vi "VGD ECL AHMI PF SubVI04.vi"(0 "SUPERIOR":T1, 1 "error in":errorcluster) -> (2 "Redondez":dbl, 3 "Analisis superior":T1(plugin-control), 4 "error out":errorcluster)   [LabVIEW 2020]
uses:
  <vilib>/vision/Image Controls.llb/IMAQ Image.ctl
  <vilib>/vision/Measure.llb/Edge Options.ctl
  <vilib>/vision/Measure.llb/Edge Polarity.ctl
  <vilib>/vision/NI_Vision_Development_Module.lvlib
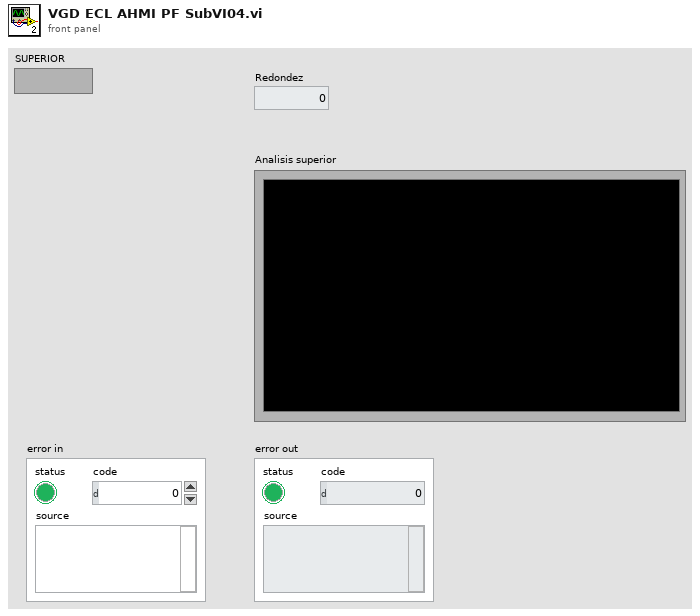
[diagram p1: front panel]
types:
  T1 = typedef "IMAQ Image.ctl" = refnum<image>
  T2 = typedef "Edge Options.ctl" = cluster{"Edge Polarity":T3, "Kernel Size":u32, "Width":u32, "Minimum Edge Strength":sgl, "Interpolation Type":enum32{"Zero Order", "Bilinear", "Quadratic", "Cubic", "Bilinear Fixed"}, "Data Processing Method":enum32{"Average", "Median"}}
  T3 = typedef "Edge Polarity.ctl" = u32
  T4 = cluster{"Search  Direction":u32, "Edge Options":T2, "Show Search Area":bool, "Show Search Lines":bool, "Show Edges Found":bool, "Show Result":bool, "Search Area Color":u32, "Search Lines Color":u32, "Edge Locations Color":u32, "Result Color":u32, "Overlay Group Name":string}
  T5 = cluster{"Process":enum16{"Get First Edge", "Get First + Last Edge", "Get All Edges", "Get Best Edge"}, "Step Size":dbl, "Max Pixel Radius":i32}
  T6 = typedef "IMAQ Circle" = cluster{"Center X":i32, "Center Y":i32, "Inner Radius":i32, "Outer Radius":i32, "Start Angle":dbl, "End Angle":dbl}
  T7 = typedef "ROI Descriptor" = cluster{"Global Rectangle":i32[], "Contours":cluster{"ID":enum32{"External", "Internal"}, "Type":u32, "Coordinates":i32[]}[]}
  T8 = cluster{"Center (Pixels)":cluster{"X":sgl, "Y":sgl}, "Radius (Pixels)":dbl, "Center (Real-World)":cluster{"X":sgl, "Y":sgl}, "Radius (Real-World)":dbl, "Roundness (Real-World)":dbl, "Average Strength":dbl, "Average SNR (dB)":dbl}
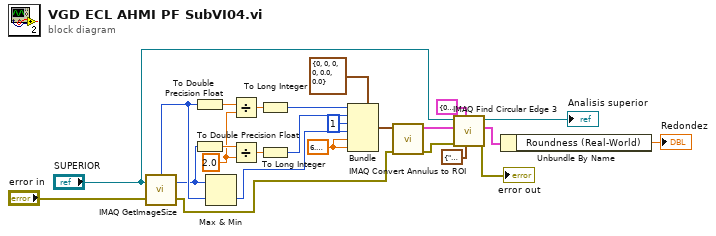
[diagram p0: block diagram]
diagram:
  w17 = 2.0 ("y")
  w20 = 6.283185307179586
  n1 = call "IMAQ GetImageSize"("Image"="SUPERIOR", "error in (no error)"="error in") -> ("Y Resolution"=w8:i32, "X Resolution"=w9:i32, "error out"=w7:errorcluster)  [unwired: 2 in]
  n2 = To Double Precision Float(number=w9) -> (double precision float=w19:dbl)
  n3 = To Double Precision Float(number=w8) -> (double precision float=w18:dbl)
  n4 = Max & Min(x=w8, y=w9) -> (min(x,y)=w12:i32)  [unwired: 1 out]
  n5 = Divide(x=w19, y=w17) -> (x/y=w16:dbl)
  n6 = Divide(x=w18, y=w17) -> (x/y=w15:dbl)
  n7 = To Long Integer(number=w16) -> (32bit integer=w14:i32)
  n8 = To Long Integer(number=w15) -> (32bit integer=w13:i32)
  n9 = Bundle(cluster=T6 {"Center X"=0, "Center Y"=0, "Inner Radius"=0, "Outer Radius"=0, "Start Angle"=0.0, "End Angle"=0.0} ("Annulus"), "Center X"=w14, "Center Y"=w13, "Inner Radius"=1, "Outer Radius"=w12, "Start Angle"=w20, "End Angle"=w20) -> (w21:T6)
  n10 = call "IMAQ Convert Annulus to ROI"("error in (no error)"=w7, "Annulus"=w21) -> ("error out"=w11:errorcluster, "ROI Descriptor"=w25:T7)  [unwired: 7 in]
  n11 = call "IMAQ Find Circular Edge 3"("Circle Fit Options"=T5 {"Process"=enum."Get First Edge", "Step Size"=3.0, "Max Pixel Radius"=3}, "Options"=T4 {"Search  Direction"=0, "Edge Options"={"Edge Polarity"=0, "Kernel Size"=3, "Width"=3, "Minimum Edge Strength"=10.0, "Interpolation Type"=enum."Bilinear Fixed", "Data Processing Method"=enum."Average"}, "Show Search Area"=FALSE, "Show Search Lines"=FALSE, "Show Edges Found"=TRUE, "Show Result"=TRUE, "Search Area Color"=65280, "Search Lines Color"=255, "Edge Locations Color"=16776960, "Result Color"=16711680, "Overlay Group Name"=""}, "error in (no error)"=w11, "ROI Descriptor"=w25, "Image"="SUPERIOR") -> ("error out"=→"error out":errorcluster, "Fitted Circle"=w4:T8, "Image Out"=→"Analisis superior":T1)  [unwired: 2 in, 2 out]
  n12 = Unbundle By Name(w4) -> ("Roundness (Real-World)"=→"Redondez":dbl)
